vi "XY to Waveform Cluster (1D).vi"(1 "X":dbl[](array[numeric]), 2 "Y":dbl[](array[numeric])) -> (5 "waveform cluster":cluster{dbl, "dx":dbl, "Y":dbl[]})   [LabVIEW 2020]
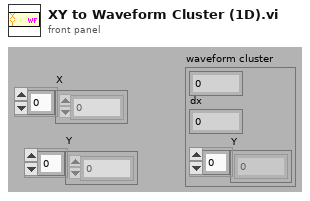
[diagram p1: front panel]
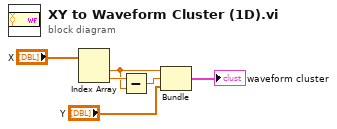
[diagram p0: block diagram]
diagram:
  n1 = Index Array(array="X") -> (element #1=w2:dbl, element #2=w3:dbl)  [unwired: 2 in]
  n2 = Subtract(x=w3, y=w2) -> (x-y=w1:dbl)
  n3 = Bundle("Numeric"=w2, w1, "Y"="Y") -> (→"waveform cluster":cluster{"Numeric":dbl, dbl, "Y":dbl[]})  [unwired: 1 in]
